vi "on-off-hist.vi"(0 "Array":i16[](array[numeric]), 1 "Data bin time":dbl format="%.2f", 2 "Threshold":sgl format="%.2f", 3 "Threshold 2":sgl format="%.2f") -> (4 "0n 2":cluster{"Axis":dbl[], "Histogram":i32[]}(graph), 5 "Avg off":dbl format="%.2f", 6 "off times":i32[](array[numeric]), 7 "Avg On":dbl format="%.2f", 8 "on times":i32[](array[numeric]), 9 "On plot 1":cluster{"Axis":dbl[], "Histogram":i32[]}(graph), 10 "Offs 0":cluster{"Axis":dbl[], "Histogram":i32[]}(graph))   [LabVIEW 2009]
uses:
  <vilib>/Analysis/NI_AALPro.lvlib
  <vilib>/Analysis/NI_AALBase.lvlib
panel:
  out "Avg off 2":dbl format="%.2f"
  out "Avg On 2":dbl format="%.2f"
  out "off times 2":i32[](array[numeric])
  out "on times 2":i32[](array[numeric])
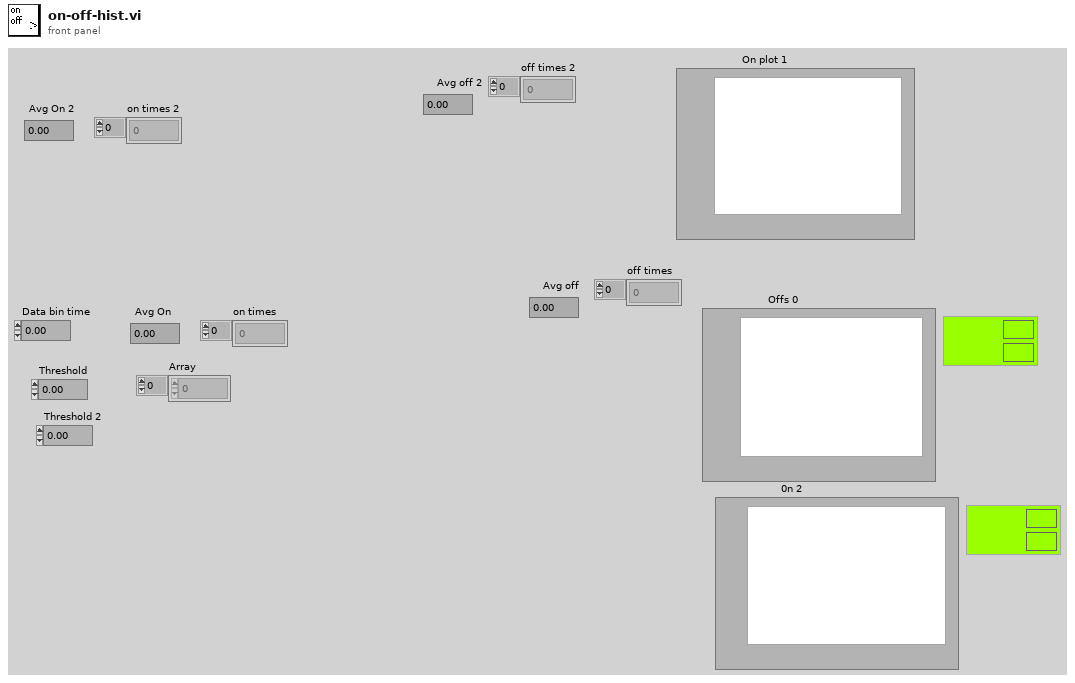
[diagram p1: front panel]
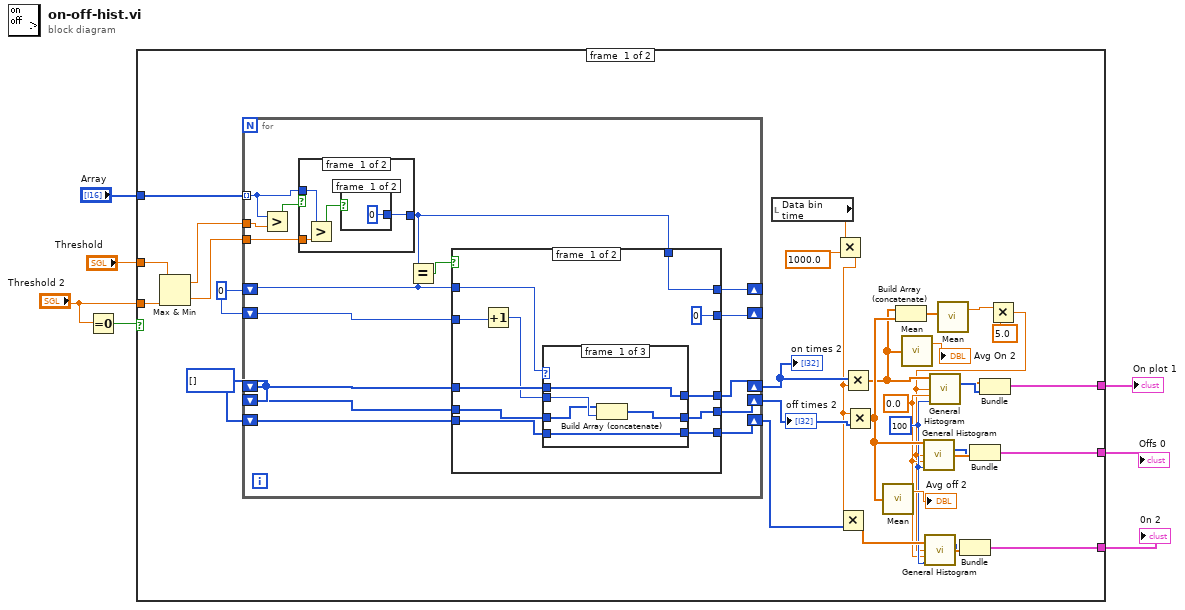
[diagram p0: block diagram]
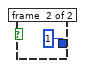
[diagram p2: hidden frame]
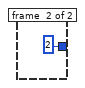
[diagram p3: hidden frame]
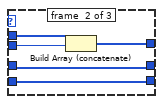
[diagram p4: hidden frame]
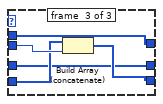
[diagram p5: hidden frame]
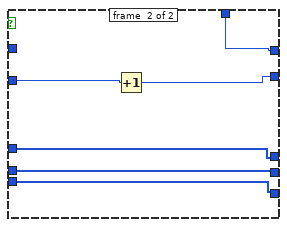
[diagram p6: hidden frame]
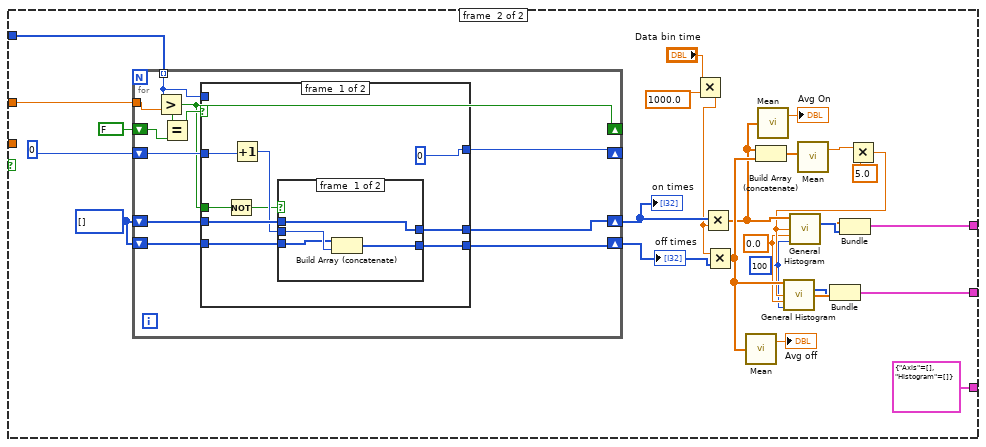
[diagram p7: hidden frame]
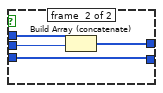
[diagram p8: hidden frame]
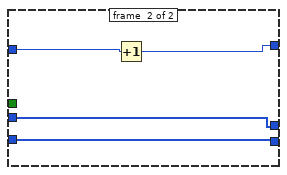
[diagram p9: hidden frame]
diagram:
  n1 = Equal To 0?(x="Threshold 2") -> (x = 0?=w6:bool)
  n2 = case shown="False" w6 {
    tunnel: "Threshold" -> [w25 w103]
    tunnel: "Threshold 2" -> [w24 _]
    tunnel: "Array" -> [w23 w104]
    tunnel: [w13 w98] -> w3
    tunnel: [w12 w97] -> w2
    tunnel: [w11 cluster{"Axis":dbl[], "Histogram":i32[]} {"Axis"=[], "Histogram"=[]}] -> w1
    frame #0 {
      w22 = 0
      w27 = i32[] []
      w15 = 0.0 ("min")
      w16 = 100 ("# bins")
      n3 = Max & Min(x=w25, y=w24) -> (max(x,y)=w10:sgl, min(x,y)=w9:sgl)
      n4 = for {
        shift-right: [w55] -> _
        shift-left: w22 -> [w56]
        shift-right: [w54] -> w29
        shift-left: w27 -> [w53]
        shift-right: [w52] -> w28
        shift-left: w27 -> [w51]
        shift-right: [w43] -> _
        shift-left: w22 -> [w45]
        tunnel: w23 -> [w48] mode=indexing
        tunnel: w9 -> [w47]
        tunnel: w10 -> [w50]
        shift-right: [w41] -> w18
        shift-left: w27 -> [w42]
        n5 = Greater?(x=w48, y=w50) -> (0:w49:bool)
        n6 = case shown="False" w49 {
          tunnel: w48 -> [w60 _]
          tunnel: w47 -> [w59 _]
          tunnel: [w57 2] -> w44
          frame #0 {
            n7 = Greater?(x=w60, y=w59) -> (0:w58:bool)
            n8 = case shown="False" w58 {
              tunnel: [0 1] -> w57
              frame #0 {
              }
              frame #1 {
              }
            }
          }
          frame #1 {
          }
        }
        n9 = Equal?(x=w44, y=w45) -> (x = y?=w46:bool)
        n10 = case shown="True" w46 {
          tunnel: w56 -> [w69 w95]
          tunnel: [0 w94] -> w55
          tunnel: [w73 w93] -> w54
          tunnel: w53 -> [w72 w93]
          tunnel: [w71 w92] -> w52
          tunnel: w51 -> [w70 w92]
          tunnel: w45 -> [w67 _]
          tunnel: w44 -> [w66 w91]
          tunnel: [w66 w91] -> w43
          tunnel: w42 -> [w65 w90]
          tunnel: [w64 w90] -> w41
          frame #0 {
            n11 = Increment(x=w69) -> (x+1=w68:i32)
            n12 = case shown="0, Default" w67 {
              tunnel: w68 -> [w78 w84 w89]
              tunnel: [w79 w83 w85] -> w73
              tunnel: w72 -> [w79 w82 w85]
              tunnel: [w77 w81 w86] -> w71
              tunnel: w70 -> [w76 w81 w86]
              tunnel: w65 -> [w75 w80 w88]
              tunnel: [w75 w80 w87] -> w64
              frame #0 {
                n13 = Build Array (concatenate)(w76, w78) -> (w77:i32[])
              }
              frame #1 {
                n14 = Build Array (concatenate)(w82, w84) -> (w83:i32[])
              }
              frame #2 {
                n15 = Build Array (concatenate)(w88, w89) -> (w87:i32[])
              }
            }
          }
          frame #1 {
            n16 = Increment(x=w95) -> (x+1=w94:i32)
          }
        }
      }
      "off times 2" <- w28
      "on times 2" <- w29
      n17 = local read "Data bin time"() -> (w8:dbl)
      n18 = Multiply(x=w8, y=1000.0) -> (x*y=w19:dbl)
      n19 = Multiply(x=w19, y=w18) -> (x*y=w17:dbl[])
      n20 = Multiply(x=w29, y=w19) -> (x*y=w37:dbl[])
      n21 = Multiply(x=w19, y=w28) -> (x*y=w40:dbl[])
      n22 = call <vilib>:"Mean.vi"("X"=w40) -> ("mean"=→"Avg off 2":dbl)  [unwired: 1 out]
      n23 = Build Array (concatenate)(w37, w40) -> (w30:dbl[])
      n24 = call <vilib>:"Mean.vi"("X"=w37) -> ("mean"=→"Avg On 2":dbl)  [unwired: 1 out]
      n25 = call <vilib>:"Mean.vi"("X"=w30) -> ("mean"=w31:dbl)  [unwired: 1 out]
      n26 = Multiply(x=w31, y=5.0) -> (x*y=w14:dbl)
      n27 = call <vilib>:"General Histogram.vi"("X"=w40, "max"=w14, "min"=w15, "# bins"=w16) -> ("Histogram"=w35:i32[], "Axis"=w36:dbl[])  [unwired: 7 in, 3 out]
      n28 = call <vilib>:"General Histogram.vi"("X"=w17, "max"=w14, "min"=w15, "# bins"=w16) -> ("Histogram"=w20:i32[], "Axis"=w21:dbl[])  [unwired: 7 in, 3 out]
      n29 = call <vilib>:"General Histogram.vi"("X"=w37, "max"=w14, "min"=w15, "# bins"=w16) -> ("Histogram"=w34:i32[], "Axis"=w33:dbl[])  [unwired: 7 in, 3 out]
      n30 = Bundle("Axis"=w21, "Histogram"=w20) -> (w11:cluster{"Axis":dbl[], "Histogram":i32[]})  [unwired: 1 in]
      n31 = Bundle("Axis"=w36, "Histogram"=w35) -> (w12:cluster{"Axis":dbl[], "Histogram":i32[]})  [unwired: 1 in]
      n32 = Bundle("Axis"=w33, "Histogram"=w34) -> (w13:cluster{"Axis":dbl[], "Histogram":i32[]})  [unwired: 1 in]
    }
    frame #1 {
      w106 = i32[] []
      w115 = 0.0 ("min")
      w114 = 100 ("# bins")
      n33 = for {
        tunnel: w104 -> [w126] mode=indexing
        shift-right: [w132] -> _
        shift-left: 0 ("Index") -> [w133]
        shift-right: [w131] -> w108
        shift-left: w106 -> [w130]
        shift-right: [w129] -> w107
        shift-left: w106 -> [w128]
        shift-right: [w123] -> _
        shift-left: FALSE -> [w125]
        tunnel: w103 -> [w127]
        n34 = Greater?(x=w126, y=w127) -> (0:w123:bool)
        n35 = Equal?(x=w123, y=w125) -> (x = y?=w124:bool)
        n36 = case shown="True" w124 {
          tunnel: w126 -> [_ _]
          tunnel: w133 -> [w137 w154]
          tunnel: [0 w153] -> w132
          tunnel: [w141 w152] -> w131
          tunnel: w130 -> [w140 w152]
          tunnel: [w139 w151] -> w129
          tunnel: w128 -> [w138 w151]
          tunnel: w123 -> [w135 _]
          frame #0 {
            n37 = Not(x=w135) -> (.not. x?=w134:bool)
            n38 = Increment(x=w137) -> (x+1=w136:i32)
            n39 = case shown="True" w134 {
              tunnel: w136 -> [w145 w150]
              tunnel: [w146 w149] -> w141
              tunnel: w140 -> [w146 w148]
              tunnel: [w144 w147] -> w139
              tunnel: w138 -> [w143 w147]
              frame #0 {
                n40 = Build Array (concatenate)(w143, w145) -> (w144:i32[])
              }
              frame #1 {
                n41 = Build Array (concatenate)(w148, w150) -> (w149:i32[])
              }
            }
          }
          frame #1 {
            n42 = Increment(x=w154) -> (x+1=w153:i32)
          }
        }
      }
      "off times" <- w107
      "on times" <- w108
      n43 = Multiply(x="Data bin time", y=1000.0) -> (x*y=w99:dbl)
      n44 = Multiply(x=w108, y=w99) -> (x*y=w119:dbl[])
      n45 = Multiply(x=w99, y=w107) -> (x*y=w122:dbl[])
      n46 = call <vilib>:"Mean.vi"("X"=w122) -> ("mean"=→"Avg off":dbl)  [unwired: 1 out]
      n47 = Build Array (concatenate)(w119, w122) -> (w109:dbl[])
      n48 = call <vilib>:"Mean.vi"("X"=w119) -> ("mean"=→"Avg On":dbl)  [unwired: 1 out]
      n49 = call <vilib>:"Mean.vi"("X"=w109) -> ("mean"=w110:dbl)  [unwired: 1 out]
      n50 = Multiply(x=w110, y=5.0) -> (x*y=w116:dbl)
      n51 = call <vilib>:"General Histogram.vi"("X"=w122, "max"=w116, "min"=w115, "# bins"=w114) -> ("Histogram"=w117:i32[], "Axis"=w118:dbl[])  [unwired: 7 in, 3 out]
      n52 = call <vilib>:"General Histogram.vi"("X"=w119, "max"=w116, "min"=w115, "# bins"=w114) -> ("Histogram"=w113:i32[], "Axis"=w112:dbl[])  [unwired: 7 in, 3 out]
      n53 = Bundle("Axis"=w118, "Histogram"=w117) -> (w97:cluster{"Axis":dbl[], "Histogram":i32[]})  [unwired: 1 in]
      n54 = Bundle("Axis"=w112, "Histogram"=w113) -> (w98:cluster{"Axis":dbl[], "Histogram":i32[]})  [unwired: 1 in]
    }
  }
  "On plot 1" <- w3
  "Offs 0" <- w2
  "0n 2" <- w1
